vi "ILABW_Load_Build.vi"() -> (2 "errorOut":string, 3 "Response":string)   [LabVIEW 2012]
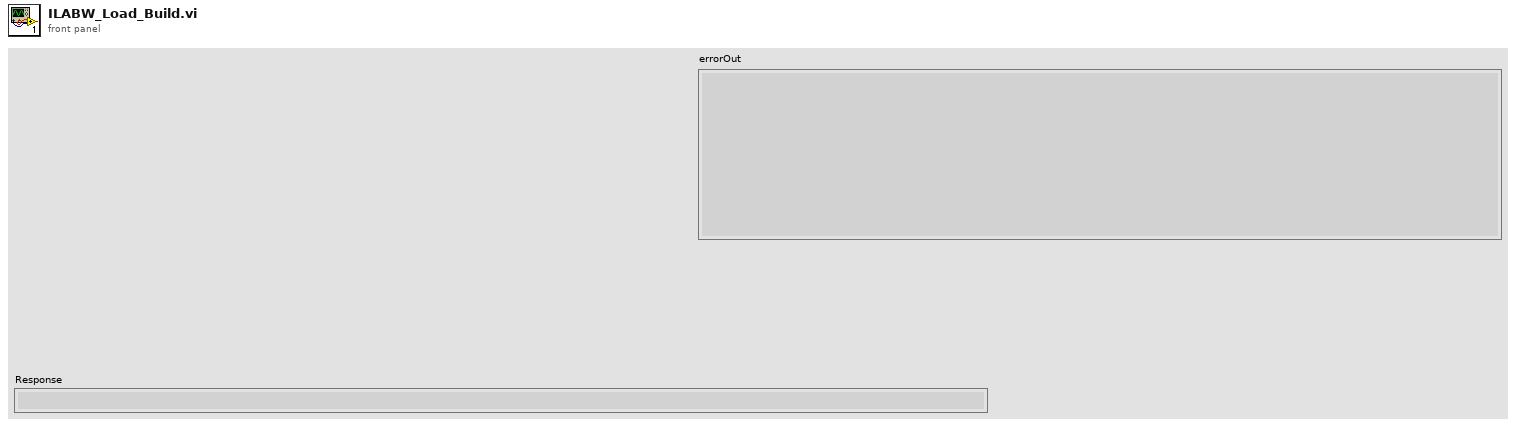
[diagram p1: front panel]
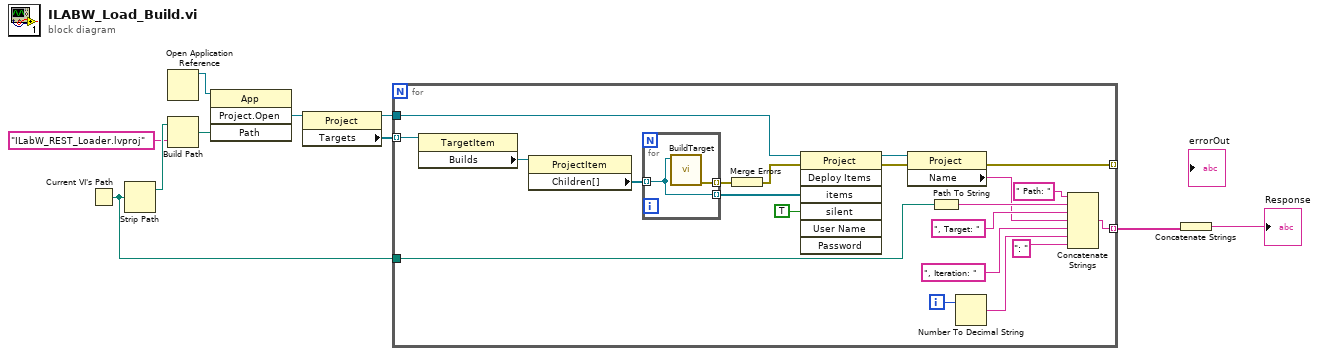
[diagram p0: block diagram]
diagram:
  n1 = Current VI's Path() -> (path=w3:path)
  n2 = Strip Path(path=w3) -> (stripped path=w10:path)  [unwired: 1 out]
  n3 = Open Application Reference() -> (3:w8:refnum<vi>)  [unwired: 4 in, 1 out]
  n4 = Build Path(base path=w10, name or relative path="ILabW_REST_Loader.lvproj") -> (appended path=w7:path)
  n5 = invoke class="App" method="Project.Open"(reference=w8, "Path"=w7) -> ("Project:Open"=w6:refnum<vi>)  [unwired: 2 in, 3 out]
  n6 = property class="Project"(reference=w6) -> (reference out=w4:refnum<vi>, "Targets"=w5:refnum<vi>[])  [unwired: 1 in, 1 out]
  n7 = for {
    tunnel: w5 -> [w31] mode=indexing
    tunnel: w4 -> [w27]
    tunnel: [w18] -> _ mode=indexing
    tunnel: [w17] -> w2 mode=indexing
    tunnel: w3 -> [w16]
    i -> [w30]
    n8 = property class="TargetItem"(reference=w31) -> ("Builds"=w26:refnum<vi>)  [unwired: 1 in, 2 out]
    n9 = property class="ProjectItem"(reference=w26) -> ("Children[]"=w24:refnum<vi>[])  [unwired: 1 in, 2 out]
    n10 = for {
      tunnel: w24 -> [w32] mode=indexing
      tunnel: [w33] -> w22 mode=indexing
      tunnel: [w32] -> w23 mode=indexing
      n11 = call <vilib>:"BuildTarget.vi"("BuildItem ref"=w32) -> ("error out"=w33:errorcluster)  [unwired: 1 in, 9 out]
    }
    n12 = Merge Errors(w22) -> (w21:errorcluster)
    n13 = invoke class="Project" method="Deploy Items"(reference=w27, error in=w21, "items"=w23, "silent"=TRUE ("Silent")) -> (reference out=w20:refnum<vi>, error out=w19:errorcluster)  [unwired: 3 in, 5 out]
    n14 = property class="Project"(reference=w20, error in=w19) -> (error out=w18:errorcluster, "Name"=w12:string)  [unwired: 1 out]
    n15 = Path To String(path=w16) -> (string=w13:string)
    n16 = Number To Decimal String(number=w30) -> (decimal integer string=w29:string)  [unwired: 1 in]
    n17 = Concatenate Strings(" Path: " ("string"), w13, ", Target: " ("string"), w12, ", Iteration: " ("string"), w29, ": " ("string")) -> (w17:string)
  }
  n18 = Concatenate Strings(w2) -> (→"Response":string)
